vi "WM Spectrum.vi"(1 "Sampling Rate":dbl format="%.2f", 2 "Time Series":dbl[](array[numeric]) format="%.2f") -> (0 "Spectra":dbl[](array[numeric]) format="%.2f")   [LabVIEW 2012]
uses:
  <vilib>/Analysis/NI_AALPro.lvlib
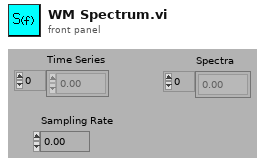
[diagram p1: front panel]
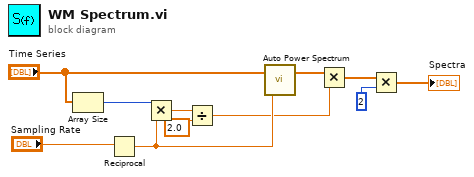
[diagram p0: block diagram]
diagram:
  n1 = Array Size(array="Time Series") -> (size(s)=w10:i32)
  n2 = Reciprocal(x="Sampling Rate") -> (1/x=w9:dbl)
  n3 = Multiply(x=w10, y=w9) -> (x*y=w7:dbl)
  n4 = Divide(x=w7, y=2.0) -> (x/y=w4:dbl)
  n5 = call <vilib>:"Auto Power Spectrum.vi"("dt"=w9, "Signal (V)"="Time Series") -> ("Power Spectrum (V^2 rms)"=w5:dbl[])  [unwired: 1 out]
  n6 = Multiply(x=w5, y=w4) -> (x*y=w2:dbl[])
  n7 = Multiply(x=w2, y=2) -> (x*y=→"Spectra":dbl[])
